vi "RandomWalk.vi"() -> ()   [LabVIEW 2020]
uses:
  <vilib>/numeric/Random Number (Range) I64.vi
  <vilib>/numeric/sub_Random U32.vi
panel:
  in  "stop":bool
  out "Random Walk":picture
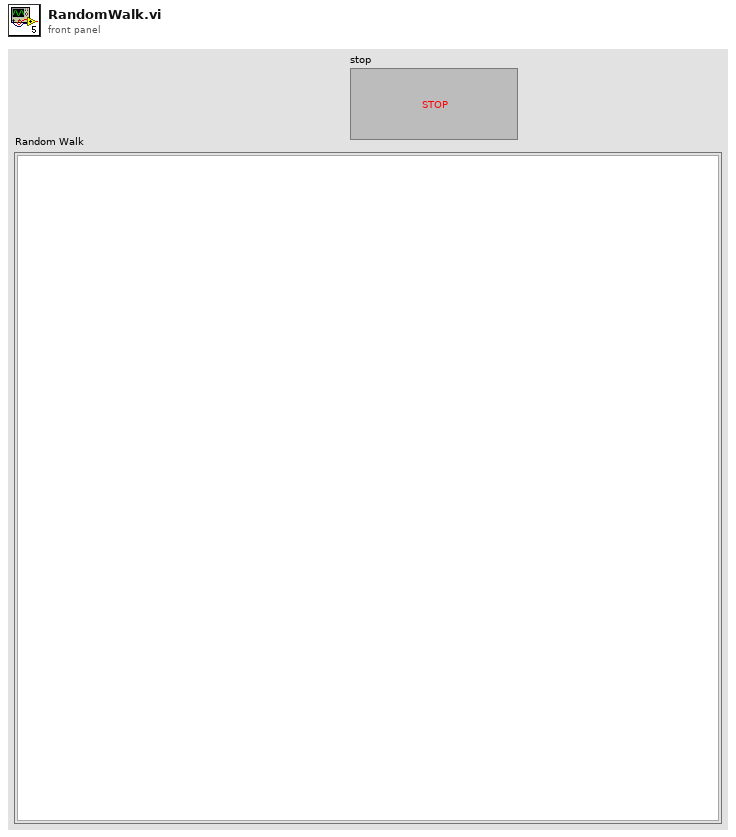
[diagram p1: front panel]
types:
  T1 = typedef "LVBoundsTypeDef.ctl" = cluster{"Width":u32, "Height":u32}
  T2 = cluster{"Width":u16, "Style":enum32{"Solid", "Dash", "Dot", "DashDot", "DashDotDot"}}
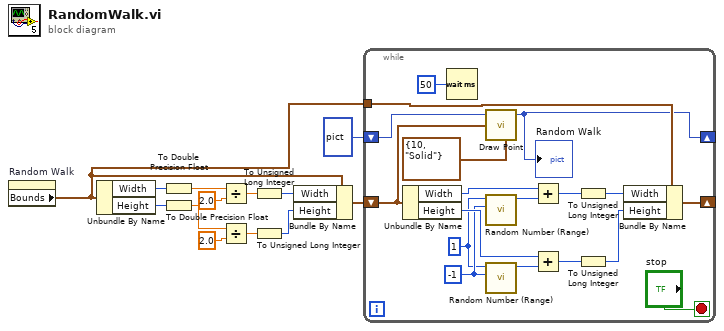
[diagram p0: block diagram]
diagram:
  n1 = property on="Random Walk" class="Pict"() -> ("Bounds"=w2:T1)  [unwired: 2 in, 2 out]
  n2 = Unbundle By Name(w2) -> ("Width"=w8:u32, "Height"=w6:u32)
  n3 = To Double Precision Float(number=w8) -> (double precision float=w7:dbl)
  n4 = To Double Precision Float(number=w6) -> (double precision float=w5:dbl)
  n5 = Divide(x=w7, y=2.0) -> (x/y=w4:dbl)
  n6 = Divide(x=w5, y=2.0) -> (x/y=w3:dbl)
  n7 = To Unsigned Long Integer(number=w4) -> (unsigned 32bit integer=w10:u32)
  n8 = To Unsigned Long Integer(number=w3) -> (unsigned 32bit integer=w9:u32)
  n9 = Bundle By Name(cluster=w2, "Width"=w10, "Height"=w9) -> (w11:T1)
  n10 = while {
    shift-right: [w27] -> _
    shift-left: w11 -> [w25]
    tunnel: w2 -> [w26]
    shift-right: [w14] -> _
    shift-left: picture data[5B] ("picture") -> [w15]
    stop <- "stop" stop-if-true
    w16 = i64 1 ("upper bound (100)")
    w17 = i64 -1 ("lower bound (-100)")
    n11 = Unbundle By Name(w25) -> ("Width"=w24:u32, "Height"=w23:u32)
    n12 = Wait (ms)(milliseconds to wait=u32 50) -> ()  [unwired: 1 out]
    n13 = call <vilib>:"Draw Point.vi"("picture"=w15, "point(x,y)"=w25, "pen"=T2 {"Width"=10, "Style"=enum."Solid"}) -> ("new picture"=w14:picture)  [unwired: 6 in]
    "Random Walk" <- w14
    n14 = call-poly <vilib>:"Random Number (Range).vi"("lower bound (-100)"=w17, "upper bound (100)"=w16) -> ("number"=w21:i64)  [unwired: 9 in]
    n15 = call-poly <vilib>:"Random Number (Range).vi"("lower bound (-100)"=w17, "upper bound (100)"=w16) -> ("number"=w22:i64)  [unwired: 9 in]
    n16 = Add(x=w24, y=w21) -> (x+y=w20:i64)
    n17 = Add(x=w23, y=w22) -> (x+y=w19:i64)
    n18 = To Unsigned Long Integer(number=w20) -> (unsigned 32bit integer=w29:u32)
    n19 = To Unsigned Long Integer(number=w19) -> (unsigned 32bit integer=w28:u32)
    n20 = Bundle By Name(cluster=w26, "Width"=w29, "Height"=w28) -> (w27:T1)
  }
